vi "isDone.vi"(8 "error in (no error)":errorcluster, 11 "PeriodicWave in":refnum<class "PeriodicWave.lvclass">) -> (0 "error out":errorcluster, 2 "isDone?":bool=TRUE, 3 "PeriodicWave out":refnum<class "PeriodicWave.lvclass">)   [LabVIEW 2015, in "PeriodicWave.lvclass"]
uses:
  PeriodicWave.lvclass
  PeriodicWave.lvclass/PeriodicWave.ctl
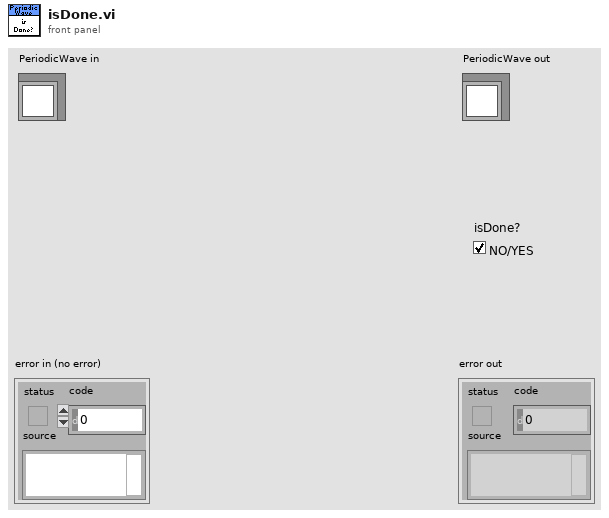
[diagram p1: front panel]
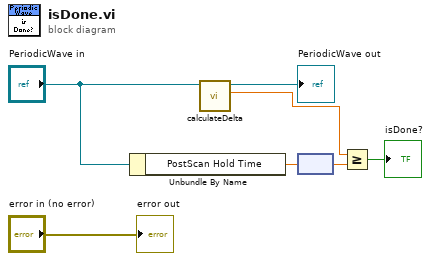
[diagram p0: block diagram]
diagram:
  n1 = Unbundle By Name("PeriodicWave in") -> ("PostScan Hold Time"=w6:dbl[unit])
  n2 = call "calculateDelta.vi"("PeriodicWave in"="PeriodicWave in") -> ("Delta Timestamp"=w3:dbl, "PeriodicWave out"=→"PeriodicWave out":refnum<class "PeriodicWave.lvclass">)  [unwired: 8 in, 1 out]
  n3 = node(w6) -> (w5:dbl)
  n4 = Greater Or Equal?(x=w3, y=w5) -> (x >= y?=→"isDone?":bool)
  "error out" <- "error in (no error)"
